vi "Value.vi"(11 "DoubleValue in":refnum<class "DoubleValue.lvclass">) -> (2 "Value":dbl)   [LabVIEW 2020, in "Futures-Examples.lvlib" / "DoubleValue.lvclass"]
uses:
  DoubleValue.lvclass
  DoubleValue.lvclass/DoubleValue.ctl
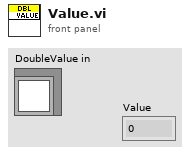
[diagram p1: front panel]
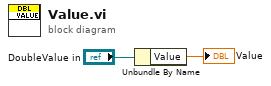
[diagram p0: block diagram]
diagram:
  n1 = Unbundle By Name("DoubleValue in") -> ("Value"=→"Value":dbl)
